vi "Buttons_Limits(Tracking_Page)-1.vi"(4 "[IN] dR max":refnum<vi>, 5 "[IN] % linearity":refnum<vi>, 6 "[IN] dR min":refnum<vi>, 7 "[IN] Min TRK L":refnum<vi>, 8 "error IN":errorcluster, 9 "[IN] Number of Frames":u32, 10 "[IN] Max angle":refnum<vi>, 11 "[IN] Closing gaps":refnum<vi>) -> (0 "error OUT":errorcluster)   [LabVIEW 2017]
doc: "Handling properties of buttons"
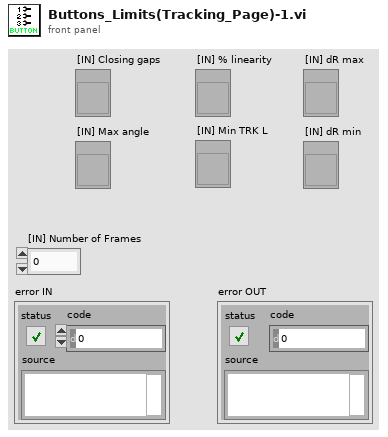
[diagram p1: front panel]
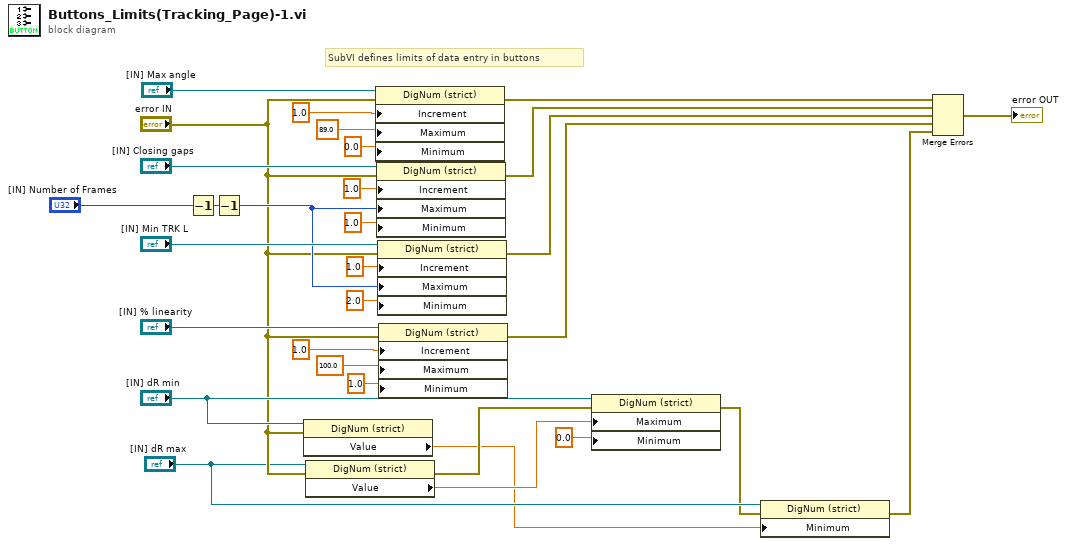
[diagram p0: block diagram]
diagram:
  # "SubVI defines limits of data entry in buttons"
  n1 = Decrement(x="[IN] Number of Frames") -> (x-1=w24:u32)
  n2 = Decrement(x=w24) -> (x-1=w20:u32)
  n3 = property on="Property Node" class="DigNum (strict)"(reference="[IN] dR min", error in="error IN") -> ("Value"=w3:dbl)  [unwired: 2 out]
  n4 = property on="Property Node" class="DigNum (strict)"(reference="[IN] dR max", error in="error IN") -> (error out=w5:errorcluster, "Value"=w8:dbl)  [unwired: 1 out]
  n5 = property on="Property Node" class="DigNum (strict)"(reference="[IN] Max angle", error in="error IN", "Increment"=1.0 ("Data Entry Limits:Increment"), "Maximum"=89.0 ("Data Entry Limits:Maximum"), "Minimum"=0.0 ("Data Entry Limits:Minimum")) -> (error out=w14:errorcluster)  [unwired: 1 out]
  n6 = property on="Property Node" class="DigNum (strict)"(reference="[IN] Closing gaps", error in="error IN", "Increment"=1.0 ("Data Entry Limits:Increment"), "Maximum"=w20, "Minimum"=1.0 ("Data Entry Limits:Minimum")) -> (error out=w13:errorcluster)  [unwired: 1 out]
  n7 = property on="Property Node" class="DigNum (strict)"(reference="[IN] Min TRK L", error in="error IN", "Increment"=1.0 ("Data Entry Limits:Increment"), "Maximum"=w20, "Minimum"=2.0 ("Data Entry Limits:Minimum")) -> (error out=w12:errorcluster)  [unwired: 1 out]
  n8 = property on="Property Node" class="DigNum (strict)"(reference="[IN] % linearity", error in="error IN", "Increment"=1.0 ("Data Entry Limits:Increment"), "Maximum"=100.0 ("Data Entry Limits:Maximum"), "Minimum"=1.0 ("Data Entry Limits:Minimum")) -> (error out=w11:errorcluster)  [unwired: 1 out]
  n9 = property on="Property Node" class="DigNum (strict)"(reference="[IN] dR min", error in=w5, "Maximum"=w8, "Minimum"=0.0 ("Data Entry Limits:Minimum")) -> (error out=w2:errorcluster)  [unwired: 1 out]
  n10 = property on="Property Node" class="DigNum (strict)"(reference="[IN] dR max", error in=w2, "Minimum"=w3) -> (error out=w1:errorcluster)  [unwired: 1 out]
  n11 = Merge Errors(w14, w13, w12, w11, w1) -> (→"error OUT":errorcluster)
